vi "Caculating avg of random numbers.vi"() -> ()   [LabVIEW 2018]
panel:
  out "random nos":dbl
  in  "n":i32
  out "avg of sum(n)":dbl
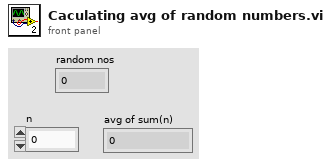
[diagram p1: front panel]
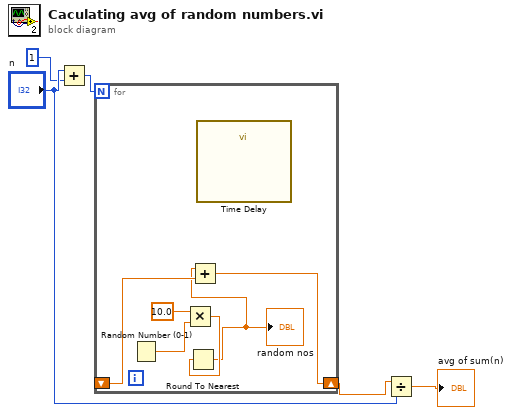
[diagram p0: block diagram]
diagram:
  n1 = Add(x="n", y=1) -> (x+y=w3:i32)
  n2 = for {
    N: w3 -> [_]
    shift-right: [w11] -> w4
    shift-left: _ -> [w10]
    n3 = Random Number (0-1)() -> (number: 0 to 1=w9:dbl)
    n4 = Multiply(x=10.0, y=w9) -> (x*y=w7:dbl)
    n5 = Round To Nearest(number=w7) -> (nearest integer value=w6:dbl)
    "random nos" <- w6
    n6 = Add(x=w6, y=w10) -> (x+y=w11:dbl)
    n7 = call "Time Delay"() -> ()  [unwired: 11 in, 1 out]
  }
  n8 = Divide(x=w4, y="n") -> (x/y=→"avg of sum(n)":dbl)
